vi "proj_main.vi"() -> ()   [LabVIEW 2020]
panel:
  out "Ilosc min dookola \nostatniego pola":i32
  out "Plansza sprawdzajaca 3":i32[][](array[numeric])
  out "Plansza sprawdzajaca 4":i32[][](array[numeric])
  out "Plansza sprawdzajaca 2":i32[][](array[numeric])
  out "Ostatnie gry":string
  in  "Table control 4":string[][](table) caption="Table control"
  in  "Sredni":bool
  out "sprawdzenie 5":i32[][](array[numeric])
  out "Plansza 5":i32[][](array[numeric])
  in  "Table control 3":string[][](table) caption="Table control"
  in  "Trudny":bool
  out "sprawdzenie 4":i32[][](array[numeric])
  out "Plansza 4":i32[][](array[numeric])
  in  "Latwy":bool
  out "sprawdzenie 3":i32[][](array[numeric])
  out "Plansza 3":i32[][](array[numeric])
  in  "Table control 2":string[][](table) caption="Table control"
  in  "Wielkosc planszy":i32
  in  "Ilosc min":i32
  out "Maksymalna ilosc \n min":i32
  out "Czas wygranej":dbl format="%<%M:%S>t"
  out "Wygrana":bool
  out "Przegrana":bool
  out "Plansza sprawdzajaca":i32[][](array[numeric])
  out "sprawdzenie":i32[][](array[numeric])
  in  "Reset":bool
  in  "Graj":bool
  in  "Table control":string[][](table)
  out "Plansza":i32[][](array[numeric])
  out "Komunikaty":string
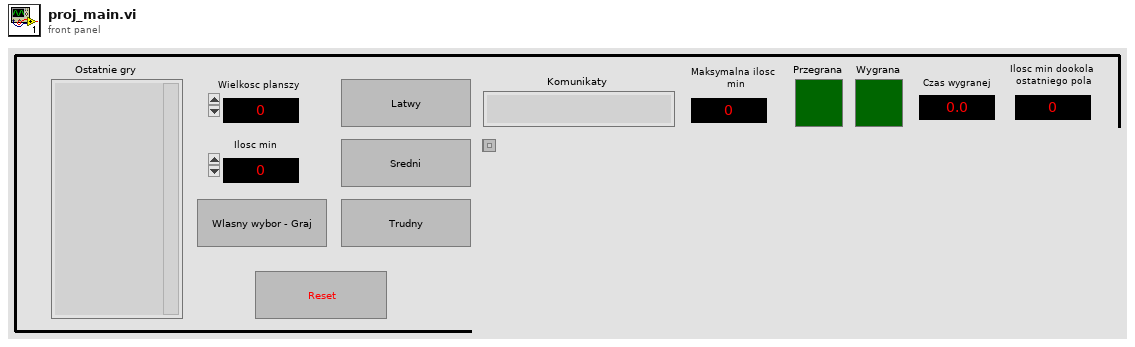
[diagram p1: front panel]
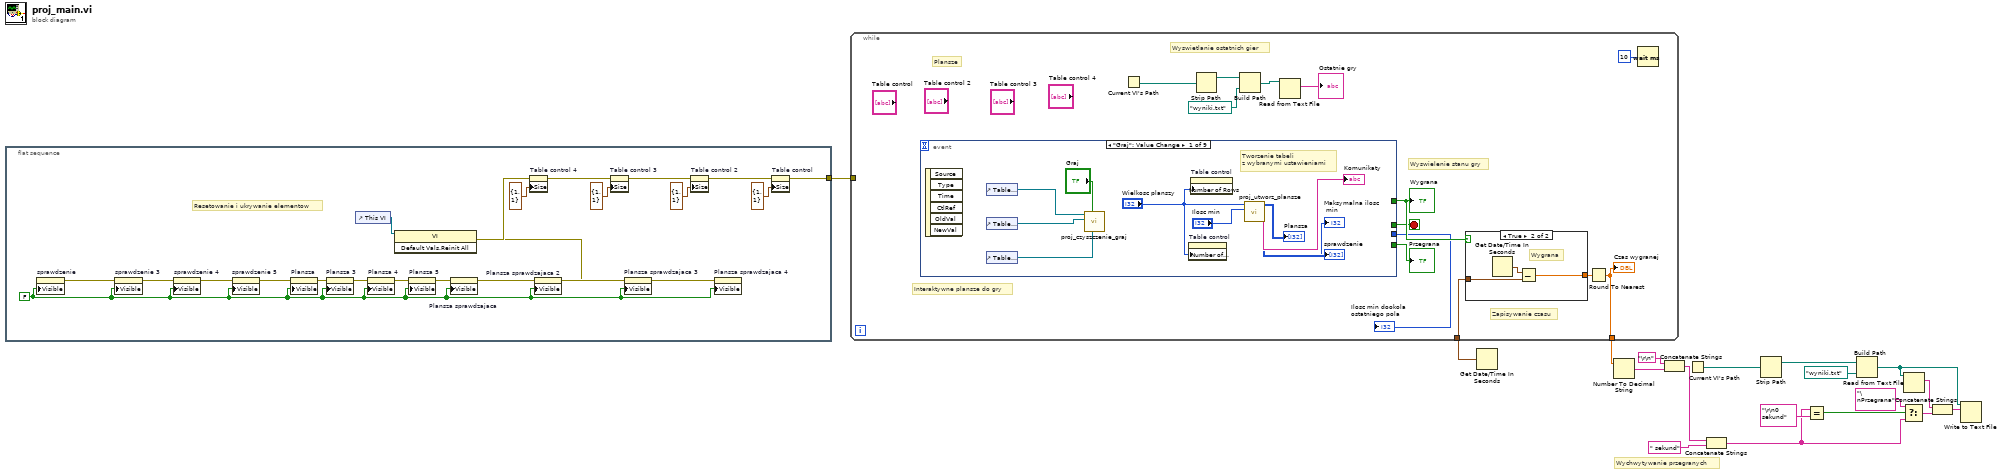
[diagram p0: block diagram]
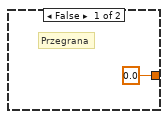
[diagram p2: hidden frame]
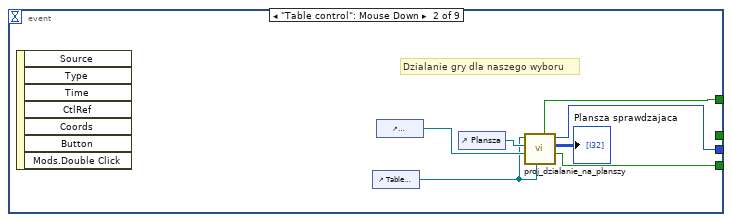
[diagram p3: hidden frame]
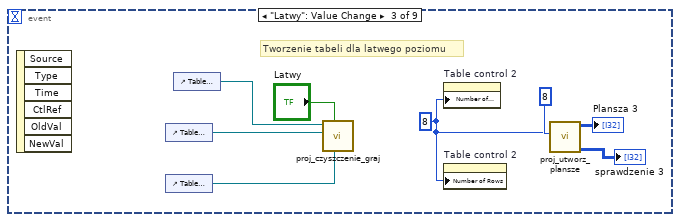
[diagram p4: hidden frame]
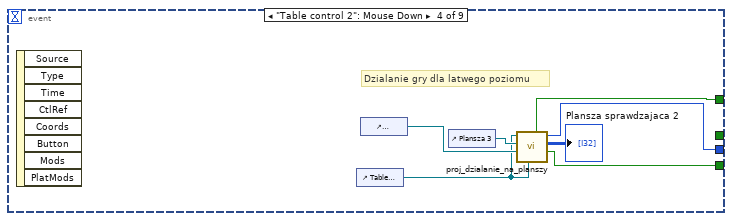
[diagram p5: hidden frame]
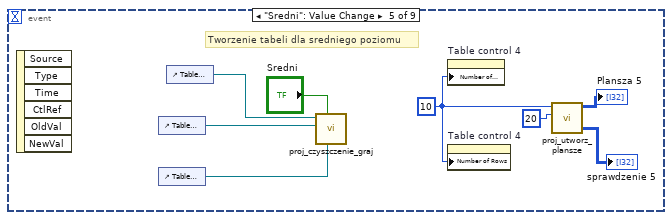
[diagram p6: hidden frame]
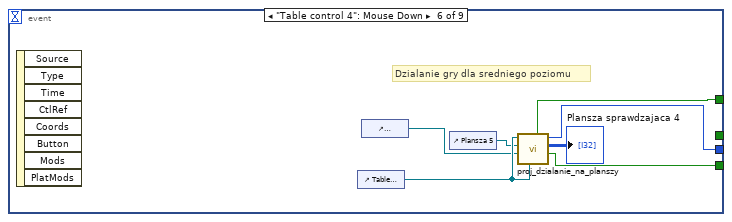
[diagram p7: hidden frame]
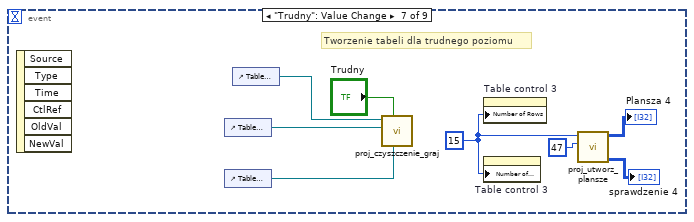
[diagram p8: hidden frame]
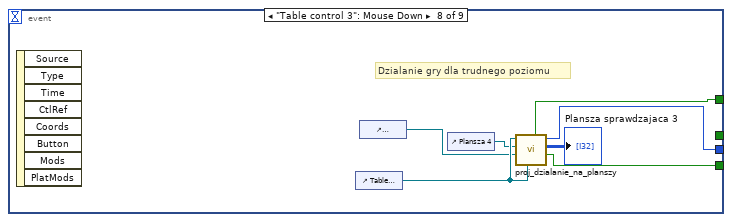
[diagram p9: hidden frame]
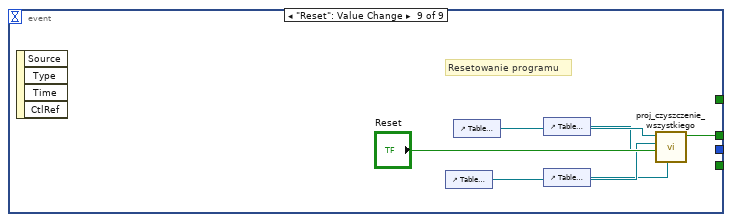
[diagram p10: hidden frame]
diagram:
  # "Wychwytywanie przegranych"
  n1 = flat-sequence {
    tunnel: [w24] -> w1
    frame #0 {
      w19 = FALSE
      # "Resetowanie i ukrywanie elementow"
      n2 = property on="sprawdzenie" class="Arr (strict)"("Visible"=w19) -> (error out=w41:errorcluster)  [unwired: 2 in, 1 out]
      n3 = property on="sprawdzenie 3" class="Arr (strict)"(error in=w41, "Visible"=w19) -> (error out=w40:errorcluster)  [unwired: 1 in, 1 out]
      n4 = property on="sprawdzenie 4" class="Arr (strict)"(error in=w40, "Visible"=w19) -> (error out=w39:errorcluster)  [unwired: 1 in, 1 out]
      n5 = property on="sprawdzenie 5" class="Arr (strict)"(error in=w39, "Visible"=w19) -> (error out=w38:errorcluster)  [unwired: 1 in, 1 out]
      n6 = property on="Plansza" class="Arr (strict)"(error in=w38, "Visible"=w19) -> (error out=w37:errorcluster)  [unwired: 1 in, 1 out]
      n7 = property on="Plansza 3" class="Arr (strict)"(error in=w37, "Visible"=w19) -> (error out=w36:errorcluster)  [unwired: 1 in, 1 out]
      n8 = control-ref of="This VI"() -> (w33:refnum<vi>)
      n9 = property on="Plansza 4" class="Arr (strict)"(error in=w36, "Visible"=w19) -> (error out=w35:errorcluster)  [unwired: 1 in, 1 out]
      n10 = property on="Plansza 5" class="Arr (strict)"(error in=w35, "Visible"=w19) -> (error out=w34:errorcluster)  [unwired: 1 in, 1 out]
      n11 = property on="Plansza sprawdzajaca" class="Arr (strict)"(error in=w34, "Visible"=w19) -> (error out=w23:errorcluster)  [unwired: 1 in, 1 out]
      n12 = property on="Plansza sprawdzajaca 2" class="Arr (strict)"(error in=w23, "Visible"=w19) -> (error out=w22:errorcluster)  [unwired: 1 in, 1 out]
      n13 = property on="Plansza sprawdzajaca 3" class="Arr (strict)"(error in=w22, "Visible"=w19) -> (error out=w21:errorcluster)  [unwired: 1 in, 1 out]
      n14 = property on="Plansza sprawdzajaca 4" class="Arr (strict)"(error in=w21, "Visible"=w19) -> (error out=w20:errorcluster)  [unwired: 1 in, 1 out]
      n15 = invoke class="VI" method="Default Vals.Reinit All"(reference=w33, error in=w20) -> (error out=w28:errorcluster)  [unwired: 1 in, 2 out]
      n16 = property on="Table control 4" class="Tbl (strict)"(error in=w28, "Size"=cluster{"Row":i32, "Column":i32} {"Row"=1, "Column"=1} ("Edit Position")) -> (error out=w27:errorcluster)  [unwired: 1 in, 1 out]
      n17 = property on="Table control 3" class="Tbl (strict)"(error in=w27, "Size"=cluster{"Row":i32, "Column":i32} {"Row"=1, "Column"=1} ("Edit Position")) -> (error out=w26:errorcluster)  [unwired: 1 in, 1 out]
      n18 = property on="Table control 2" class="Tbl (strict)"(error in=w26, "Size"=cluster{"Row":i32, "Column":i32} {"Row"=1, "Column"=1} ("Edit Position")) -> (error out=w25:errorcluster)  [unwired: 1 in, 1 out]
      n19 = property on="Table control" class="Tbl (strict)"(error in=w25, "Size"=cluster{"Row":i32, "Column":i32} {"Row"=1, "Column"=1} ("Edit Position")) -> (error out=w24:errorcluster)  [unwired: 1 in, 1 out]
    }
  }
  n20 = Get Date/Time In Seconds() -> (seconds since 1Jan1904=w18:timestamp)
  n21 = while {
    tunnel: w18 -> [w54]
    tunnel: [w51] -> w12
    tunnel: w1 -> [_]
    stop <- w42 stop-if-true
    # "Plansze"
    # "Interaktywne plansze do gry"
    # "Wyswielenie stanu gry"
    # "Zapisywanie czasu"
    # "Wyswietlanie ostatnich gier"
    n22 = event shown="[0] \"Graj\": Value Change" {
      selector: _ -> [_ _ _ _ _ _ _ _ _]
      dyn-events: _ -> [_ _ _ _ _ _ _ _ _]
      timeout: _ -> [_ _ _ _ _ _ _ _ _]
      tunnel: [_ _ _ _ _ _ _ _ w125] -> w42
      tunnel: [_ w75 _ w85 _ w100 _ w116 _] -> w45
      tunnel: [_ w74 _ w84 _ w99 _ w114 _] -> w52
      tunnel: [_ w69 _ w86 _ w101 _ w115 _] -> w43
      event "Graj": Value Change {
        # "Tworzenie tabeli \nz wybranymi ustawieniami"
        n23 = event-data() -> ()  [unwired: 1 in, 6 out]
        n24 = control-ref of="Table control 2"() -> (w61:refnum<vi>)
        n25 = control-ref of="Table control 3"() -> (w60:refnum<vi>)
        n26 = control-ref of="Table control 4"() -> (w59:refnum<vi>)
        n27 = call "proj_czyszczenie_graj.vi"("Table control 4"=w59, "Przycisk"="Graj", "Table control 2"=w60, "Table control 1"=w61) -> ()  [unwired: 8 in]
        n28 = property on="Table control" class="Tbl (strict)"("Number of Columns"="Wielkosc planszy") -> ()  [unwired: 2 in, 2 out]
        n29 = property on="Table control" class="Tbl (strict)"("Number of Rows"="Wielkosc planszy") -> ()  [unwired: 2 in, 2 out]
        n30 = call "proj_utworz_plansze.vi"("Ilosc min"="Ilosc min", "Wielkosc planszy"="Wielkosc planszy") -> ("initialized array"=→"sprawdzenie":i32[][], "Maksymalna ilosc \nmin dla danej \nwielkosci planszy"=→"Maksymalna ilosc \n min":i32, "Komunikaty"=→"Komunikaty":string, "Plansza"=→"Plansza":i32[][])  [unwired: 6 in]
      }
      event "Table control": Mouse Down {
        # "Dzialanie gry dla naszego wyboru"
        n31 = event-data() -> ()  [unwired: 1 in, 7 out]
        n32 = control-ref of="Table control"() -> (w70:refnum<vi>)
        n33 = control-ref of="sprawdzenie"() -> (w72:refnum<vi>)
        n34 = control-ref of="Plansza"() -> (w73:refnum<vi>)
        n35 = call "proj_dzialanie_na_planszy.vi"("Table control"=w70, "Tabela sprawdzajaca"=w72, "Plansza gry"=w73, "Table in"=w70) -> ("Przegrana"=w74:bool, "Plansza sprawdzajaca"=→"Plansza sprawdzajaca":i32[][], "Ilosc min dookola pola"=w69:i32, "Wygrana"=w75:bool)  [unwired: 3 in, 1 out]
      }
      event "Latwy": Value Change {
        w80 = 8 ("Ilosc min")
        # "Tworzenie tabeli dla latwego poziomu"
        n36 = event-data() -> ()  [unwired: 1 in, 6 out]
        n37 = control-ref of="Table control 3"() -> (w77:refnum<vi>)
        n38 = control-ref of="Table control 4"() -> (w76:refnum<vi>)
        n39 = control-ref of="Table control"() -> (w78:refnum<vi>)
        n40 = call "proj_czyszczenie_graj.vi"("Table control 4"=w76, "Przycisk"="Latwy", "Table control 2"=w77, "Table control 1"=w78) -> ()  [unwired: 8 in]
        n41 = property on="Table control 2" class="Tbl (strict)"("Number of Columns"=w80) -> ()  [unwired: 2 in, 2 out]
        n42 = property on="Table control 2" class="Tbl (strict)"("Number of Rows"=w80) -> ()  [unwired: 2 in, 2 out]
        n43 = call "proj_utworz_plansze.vi"("Ilosc min"=8, "Wielkosc planszy"=w80) -> ("initialized array"=→"sprawdzenie 3":i32[][], "Plansza"=→"Plansza 3":i32[][])  [unwired: 6 in, 2 out]
      }
      event "Table control 2": Mouse Down {
        # "Dzialanie gry dla latwego poziomu"
        n44 = event-data() -> ()  [unwired: 1 in, 8 out]
        n45 = control-ref of="Table control 2"() -> (w87:refnum<vi>)
        n46 = control-ref of="sprawdzenie 3"() -> (w89:refnum<vi>)
        n47 = control-ref of="Plansza 3"() -> (w90:refnum<vi>)
        n48 = call "proj_dzialanie_na_planszy.vi"("Table control"=w87, "Tabela sprawdzajaca"=w89, "Plansza gry"=w90, "Table in"=w87) -> ("Przegrana"=w84:bool, "Plansza sprawdzajaca"=→"Plansza sprawdzajaca 2":i32[][], "Ilosc min dookola pola"=w86:i32, "Wygrana"=w85:bool)  [unwired: 3 in, 1 out]
      }
      event "Sredni": Value Change {
        w95 = 10 ("Ilosc min")
        # "Tworzenie tabeli dla sredniego poziomu"
        n49 = event-data() -> ()  [unwired: 1 in, 6 out]
        n50 = control-ref of="Table control 2"() -> (w92:refnum<vi>)
        n51 = control-ref of="Table control 3"() -> (w91:refnum<vi>)
        n52 = control-ref of="Table control"() -> (w93:refnum<vi>)
        n53 = call "proj_czyszczenie_graj.vi"("Table control 4"=w91, "Przycisk"="Sredni", "Table control 2"=w92, "Table control 1"=w93) -> ()  [unwired: 8 in]
        n54 = property on="Table control 4" class="Tbl (strict)"("Number of Columns"=w95) -> ()  [unwired: 2 in, 2 out]
        n55 = property on="Table control 4" class="Tbl (strict)"("Number of Rows"=w95) -> ()  [unwired: 2 in, 2 out]
        n56 = call "proj_utworz_plansze.vi"("Ilosc min"=20, "Wielkosc planszy"=w95) -> ("initialized array"=→"sprawdzenie 5":i32[][], "Plansza"=→"Plansza 5":i32[][])  [unwired: 6 in, 2 out]
      }
      event "Table control 4": Mouse Down {
        # "Dzialanie gry dla sredniego poziomu"
        n57 = event-data() -> ()  [unwired: 1 in, 8 out]
        n58 = control-ref of="Table control 4"() -> (w105:refnum<vi>)
        n59 = control-ref of="sprawdzenie 5"() -> (w104:refnum<vi>)
        n60 = control-ref of="Plansza 5"() -> (w103:refnum<vi>)
        n61 = call "proj_dzialanie_na_planszy.vi"("Table control"=w105, "Tabela sprawdzajaca"=w104, "Plansza gry"=w103, "Table in"=w105) -> ("Przegrana"=w99:bool, "Plansza sprawdzajaca"=→"Plansza sprawdzajaca 4":i32[][], "Ilosc min dookola pola"=w101:i32, "Wygrana"=w100:bool)  [unwired: 3 in, 1 out]
      }
      event "Trudny": Value Change {
        w110 = 15 ("Ilosc min")
        # "Tworzenie tabeli dla trudnego poziomu"
        n62 = event-data() -> ()  [unwired: 1 in, 6 out]
        n63 = control-ref of="Table control 2"() -> (w109:refnum<vi>)
        n64 = control-ref of="Table control 4"() -> (w107:refnum<vi>)
        n65 = control-ref of="Table control"() -> (w108:refnum<vi>)
        n66 = call "proj_czyszczenie_graj.vi"("Table control 4"=w107, "Przycisk"="Trudny", "Table control 2"=w109, "Table control 1"=w108) -> ()  [unwired: 8 in]
        n67 = property on="Table control 3" class="Tbl (strict)"("Number of Rows"=w110) -> ()  [unwired: 2 in, 2 out]
        n68 = property on="Table control 3" class="Tbl (strict)"("Number of Columns"=w110) -> ()  [unwired: 2 in, 2 out]
        n69 = call "proj_utworz_plansze.vi"("Ilosc min"=47, "Wielkosc planszy"=w110) -> ("initialized array"=→"sprawdzenie 4":i32[][], "Plansza"=→"Plansza 4":i32[][])  [unwired: 6 in, 2 out]
      }
      event "Table control 3": Mouse Down {
        # "Dzialanie gry dla trudnego poziomu"
        n70 = event-data() -> ()  [unwired: 1 in, 8 out]
        n71 = control-ref of="Table control 3"() -> (w120:refnum<vi>)
        n72 = control-ref of="sprawdzenie 4"() -> (w119:refnum<vi>)
        n73 = control-ref of="Plansza 4"() -> (w118:refnum<vi>)
        n74 = call "proj_dzialanie_na_planszy.vi"("Table control"=w120, "Tabela sprawdzajaca"=w119, "Plansza gry"=w118, "Table in"=w120) -> ("Przegrana"=w114:bool, "Plansza sprawdzajaca"=→"Plansza sprawdzajaca 3":i32[][], "Ilosc min dookola pola"=w115:i32, "Wygrana"=w116:bool)  [unwired: 3 in, 1 out]
      }
      event "Reset": Value Change {
        # "Resetowanie programu"
        n75 = event-data() -> ()  [unwired: 1 in, 4 out]
        n76 = control-ref of="Table control 2"() -> (w123:refnum<vi>)
        n77 = control-ref of="Table control"() -> (w124:refnum<vi>)
        n78 = control-ref of="Table control 3"() -> (w122:refnum<vi>)
        n79 = control-ref of="Table control 4"() -> (w121:refnum<vi>)
        n80 = call "proj_czyszczenie_wszystkiego.vi"("Table control 4"=w121, "Reset"="Reset", "Table control 3"=w122, "Table control 2"=w123, "Table control 1"=w124) -> ("Boolean"=w125:bool)  [unwired: 6 in]
      }
    }
    "Wygrana" <- w45
    "Przegrana" <- w52
    "Ilosc min dookola \nostatniego pola" <- w43
    n81 = Current VI's Path() -> (path=w49:path)
    n82 = Strip Path(path=w49) -> (stripped path=w48:path)  [unwired: 1 out]
    n83 = Build Path(base path=w48, name or relative path=path "wyniki.txt") -> (appended path=w47:path)
    n84 = Read from Text File(file (use dialog)=w47) -> (text=→"Ostatnie gry":string)  [unwired: 3 in, 3 out]
    n85 = case shown="True" w45 {
      tunnel: [0.0 w58] -> w53
      tunnel: w54 -> [_ w56]
      frame False {
        # "Przegrana"
      }
      frame True {
        # "Wygrana"
        n86 = Get Date/Time In Seconds() -> (seconds since 1Jan1904=w57:timestamp)
        n87 = Subtract(x=w57, y=w56) -> (x-y=w58:dbl)
      }
    }
    n88 = Round To Nearest(number=w53) -> (nearest integer value=w51:dbl)
    "Czas wygranej" <- w51
    n89 = Wait (ms)(milliseconds to wait=u32 10) -> ()  [unwired: 1 out]
  }
  n90 = Number To Decimal String(number=w12) -> (decimal integer string=w10:string)  [unwired: 1 in]
  n91 = Concatenate Strings("\r\n", w10) -> (w9:string)
  n92 = Current VI's Path() -> (path=w14:path)
  n93 = Concatenate Strings(w9, " sekund" ("string")) -> (w2:string)
  n94 = Strip Path(path=w14) -> (stripped path=w15:path)  [unwired: 1 out]
  n95 = Equal?(x=w2, y="\r\n0 sekund") -> (x = y?=w5:bool)
  n96 = Build Path(base path=w15, name or relative path=path "wyniki.txt") -> (appended path=w17:path)
  n97 = Read from Text File(file (use dialog)=w17) -> (text=w16:string)  [unwired: 3 in, 3 out]
  n98 = Select(t="\nPrzegrana", s=w5, f=w2) -> (s? t:f=w3:string)
  n99 = Concatenate Strings(w16, w3) -> (w7:string)
  n100 = Write to Text File(file (use dialog)=w17, text=w7) -> ()  [unwired: 2 in, 3 out]
